vi "Main.vi"() -> ()   [LabVIEW 2014]
uses:
  Enum State Typedef.ctl
  <vilib>/Utility/error.llb/DialogType.ctl
  <vilib>/_DAQmxBase/Internals/DAQmxBase Create Channel (AI-Voltage-Basic).vi
  <vilib>/_DAQmxBase/Internals/DAQmxBase Timing (Sample Clock).vi
  <vilib>/_DAQmxBase/Internals/DAQmxBase Read (Analog 2D DBL NChan NSamp).vi
  <vilib>/Utility/file.llb/Write To Spreadsheet File (DBL).vi
panel:
  out "size(s) 2":i32
  out "State":T1
  in  "Clear Display":bool
  in  "Preview Button":bool
  out "size(s)":i32
  in  "pH":dbl
  in  "Conductivity (mS)":dbl
  out "Iterations Recorded":i32
  in  "Recording Time (seconds)":dbl
  in  "Sample Rate":i32=1000
  in  "physical channels":tag
  in  "Stop Button":bool
  out "Waveform Chart":waveform(dbl)(graph)
  in  "High Pass Filter":enum16{"500", "1k", "5k", "10k", "20k"}(ring)
  in  "Low Pass Filter":enum16{"0.1", "1.0", "10", "100", "300"}(ring)
  in  "Gain":enum16{"x100", "x1000", "x10k"}(ring)
  in  "Notch Filter":bool
  in  "Amplifier Model":u16(ring) items=["Select a Model", "AM 1700", "BMA 200"]
  in  "AC/DC Switch":bool
  in  "Temperature (deg C)":dbl
  in  "User Comments":string
  out "Start Time hr/min":string
  out "Date mm/dd/yy":string
  in  "Species":string
  in  "Exit Button":bool
  in  "Record Button":bool
  # "MSU EFISH Lab Single Channel Electronic Pulse Recorder"
  # "Must enter numbers into here before you run"
  # "Blue for On\nOrange for Off"
  # "DC"
  # "AC"
  # "Blue for AC and Orange for DC"
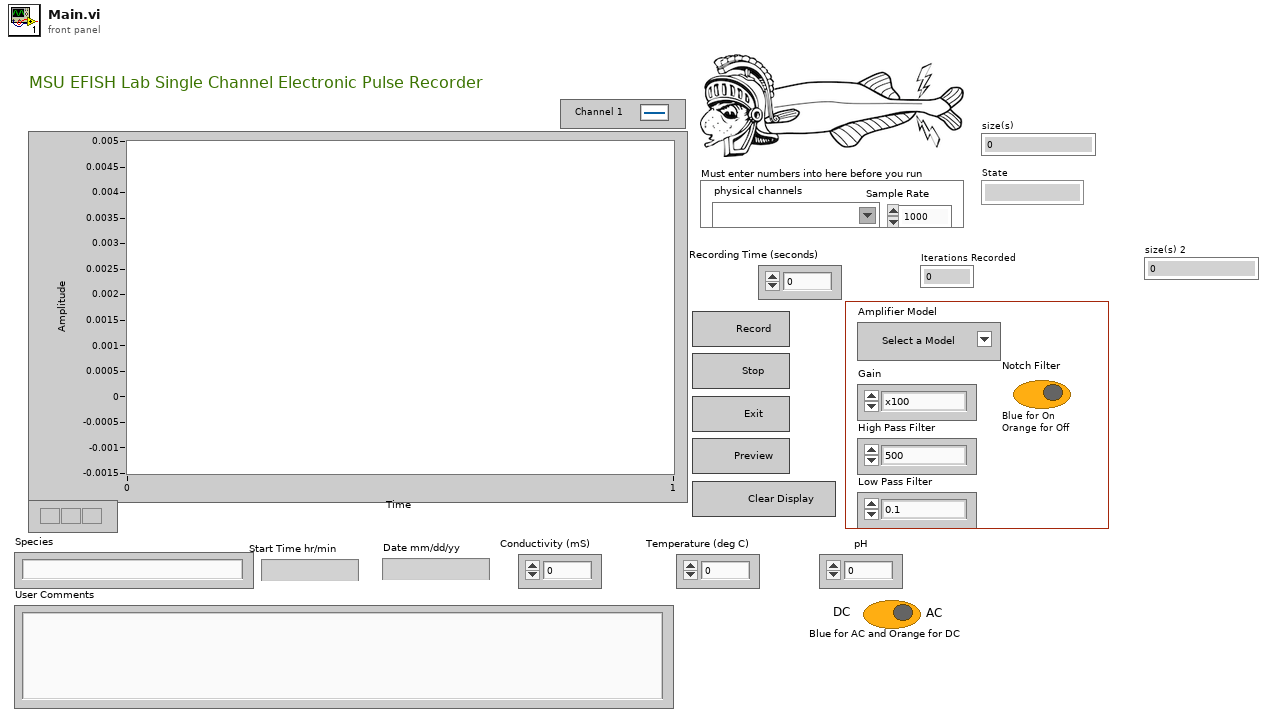
[diagram p1: front panel]
types:
  T1 = typedef "Enum State Typedef.ctl" = enum16{"", "Prepreview Handling", "Clear Display", "Preview Data", "Stop", "Exit", "Record", "Create File"}
  T2 = typedef "DialogType.ctl" = u16
  T3 = cluster{"High Pass Filter":enum16{"500", "1k", "5k", "10k", "20k"}, "Gain":enum16{"x100", "x1000", "x10k"}, "Low Pass Filter":enum16{"0.1", "1.0", "10", "100", "300"}, "Amplifier Model":u16, "Notch Filter":bool, "AC/DC Switch":bool, "Temperature (deg C)":dbl, "Conductivity (mS)":dbl, "pH":dbl, "User Comments":string, "Species":string}
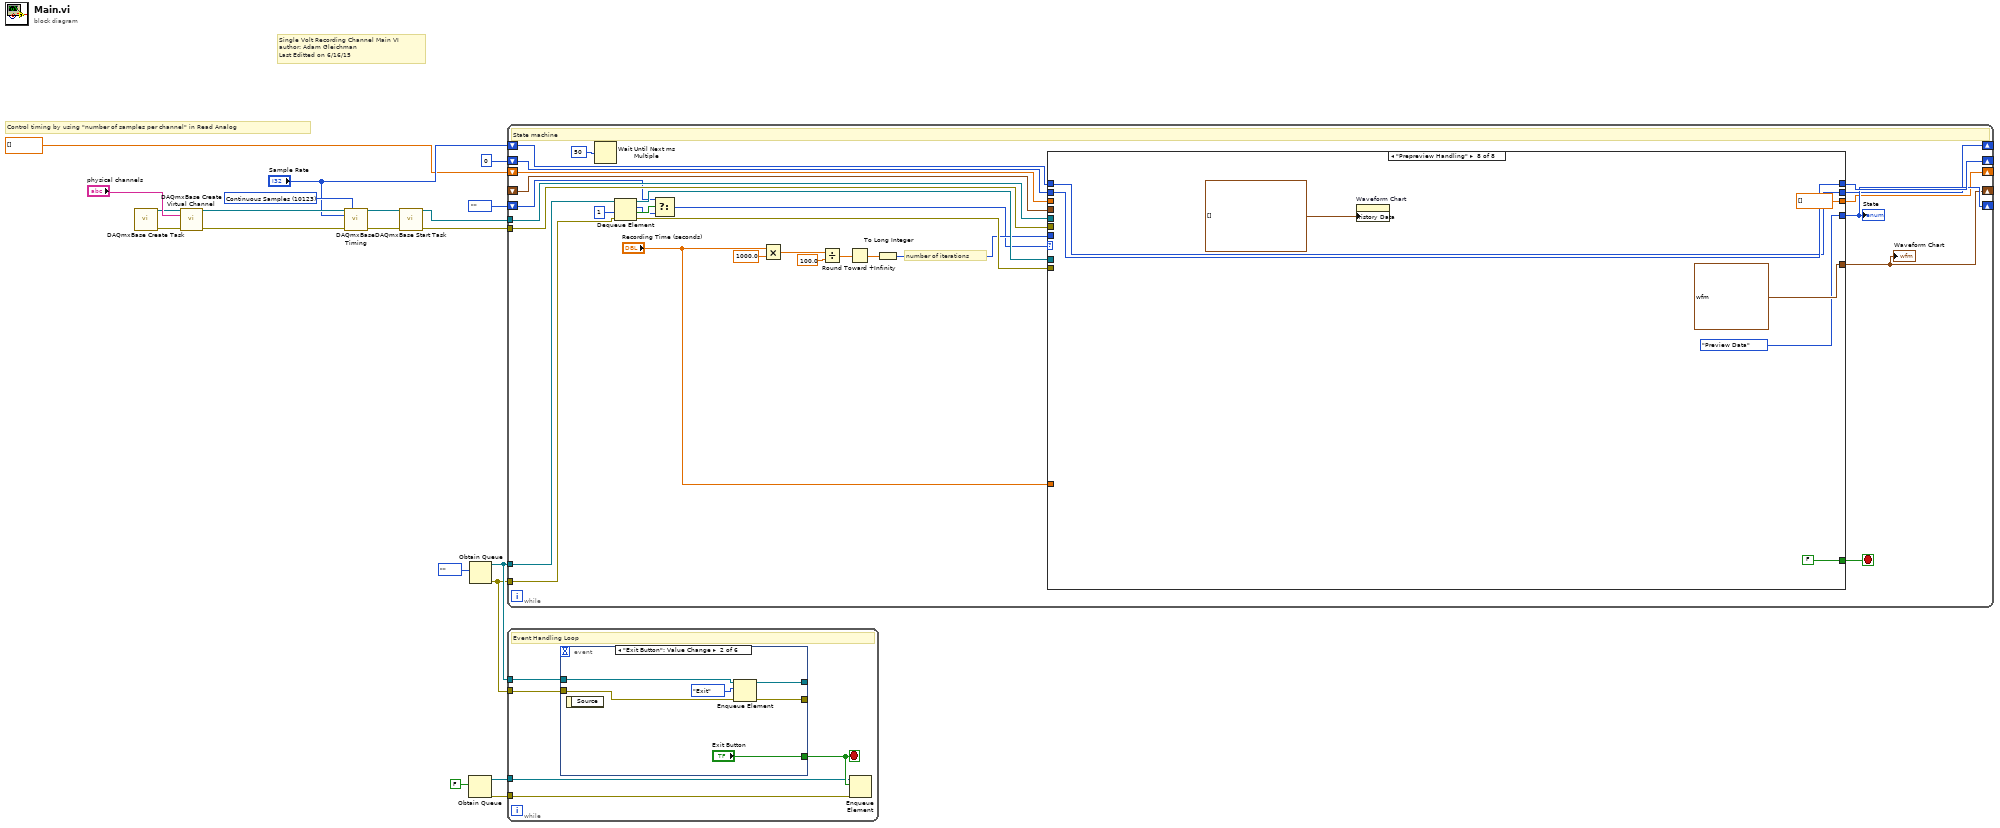
[diagram p0: block diagram]
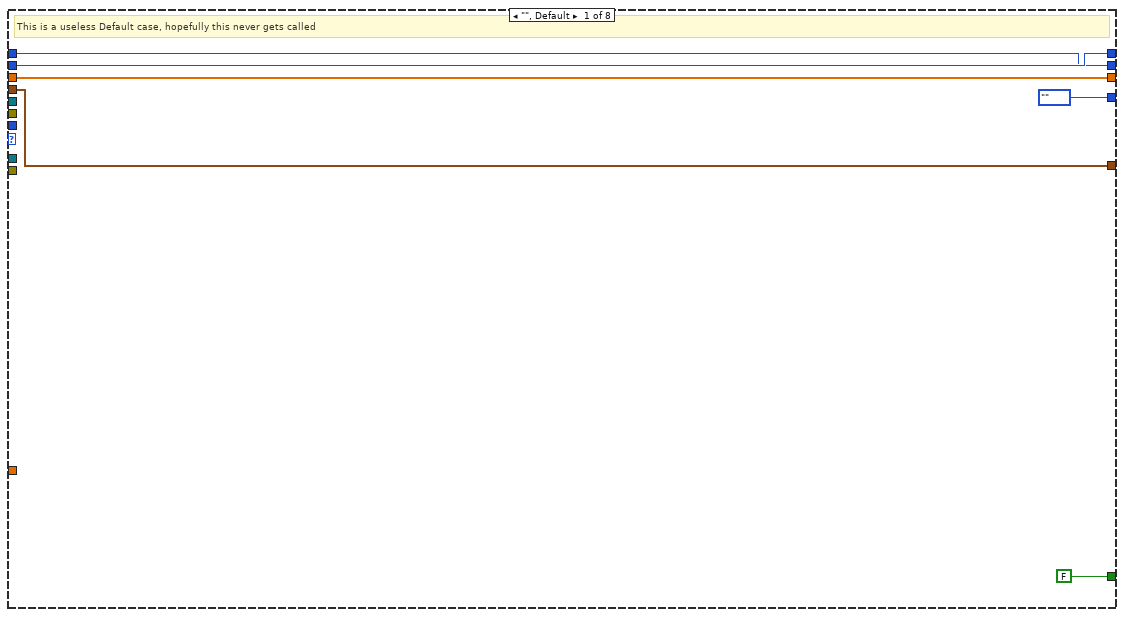
[diagram p2: hidden frame]
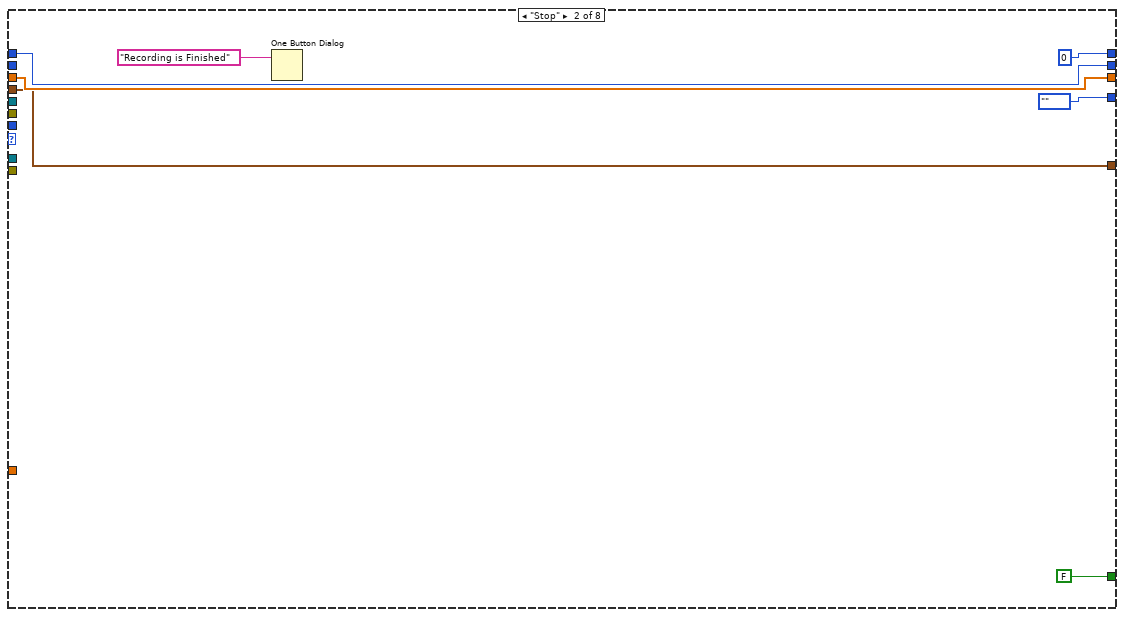
[diagram p3: hidden frame]
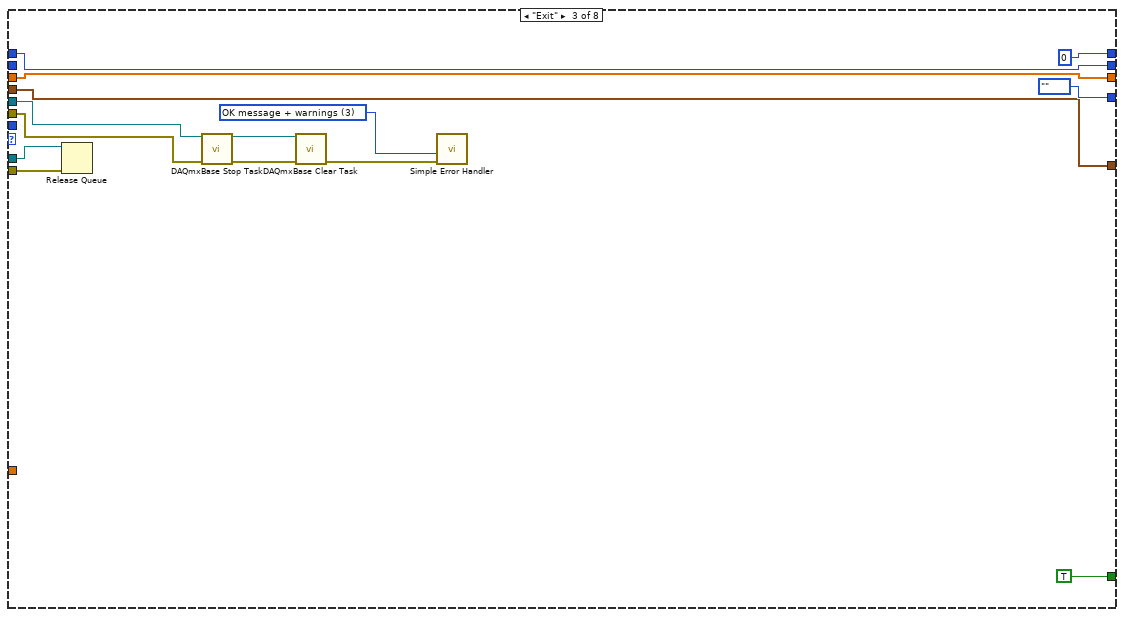
[diagram p4: hidden frame]
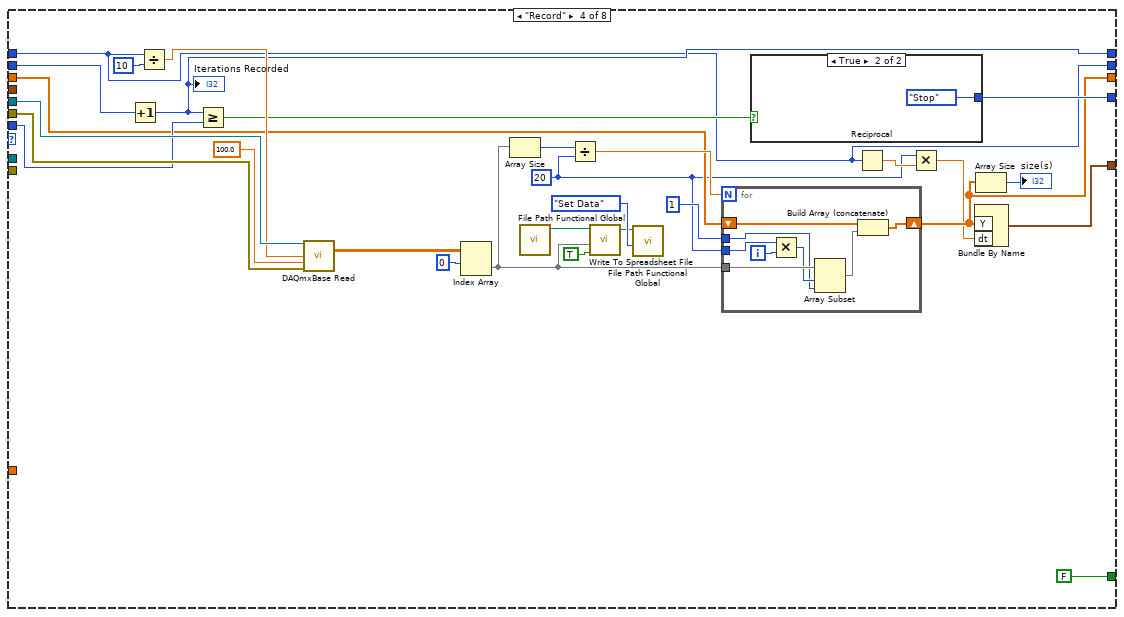
[diagram p5: hidden frame]
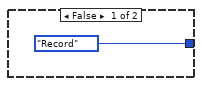
[diagram p6: hidden frame]
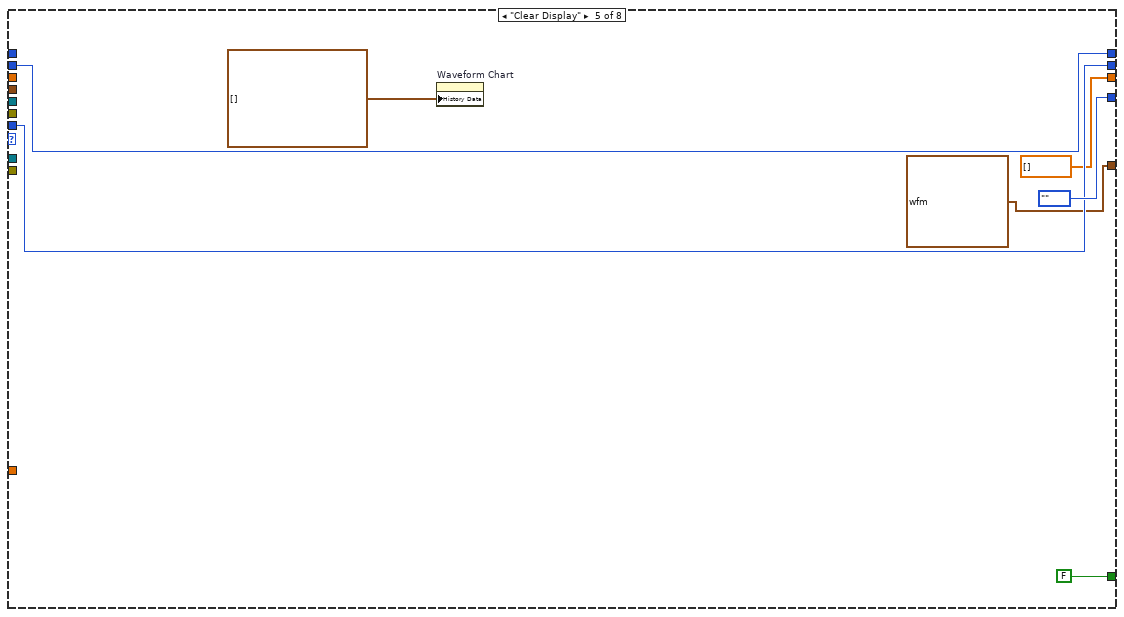
[diagram p7: hidden frame]
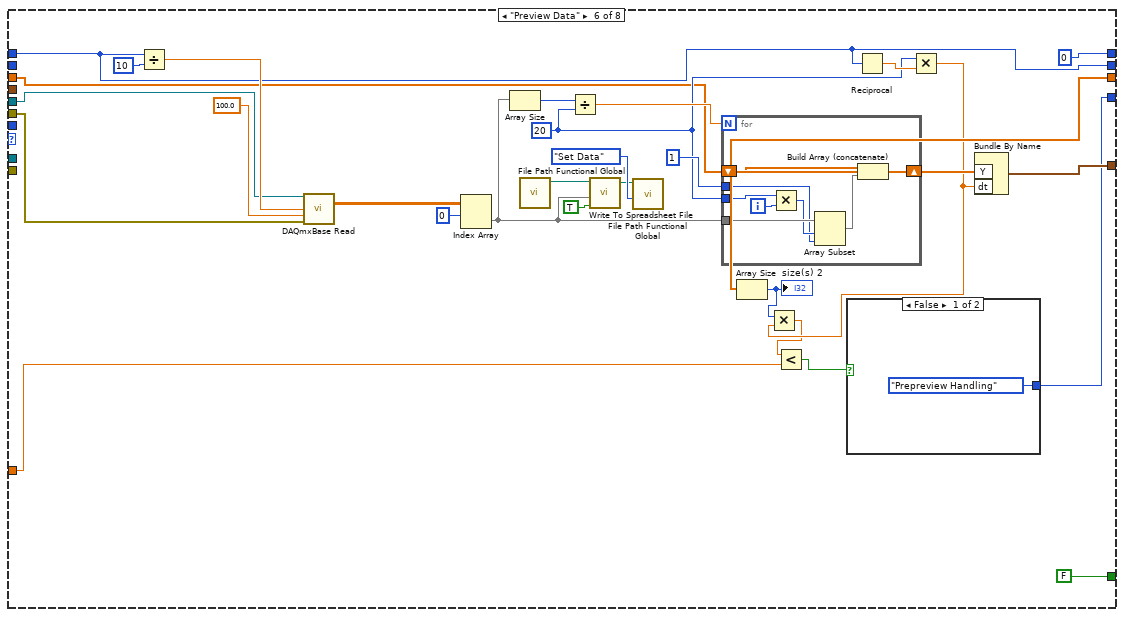
[diagram p8: hidden frame]
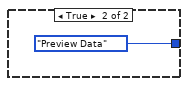
[diagram p9: hidden frame]
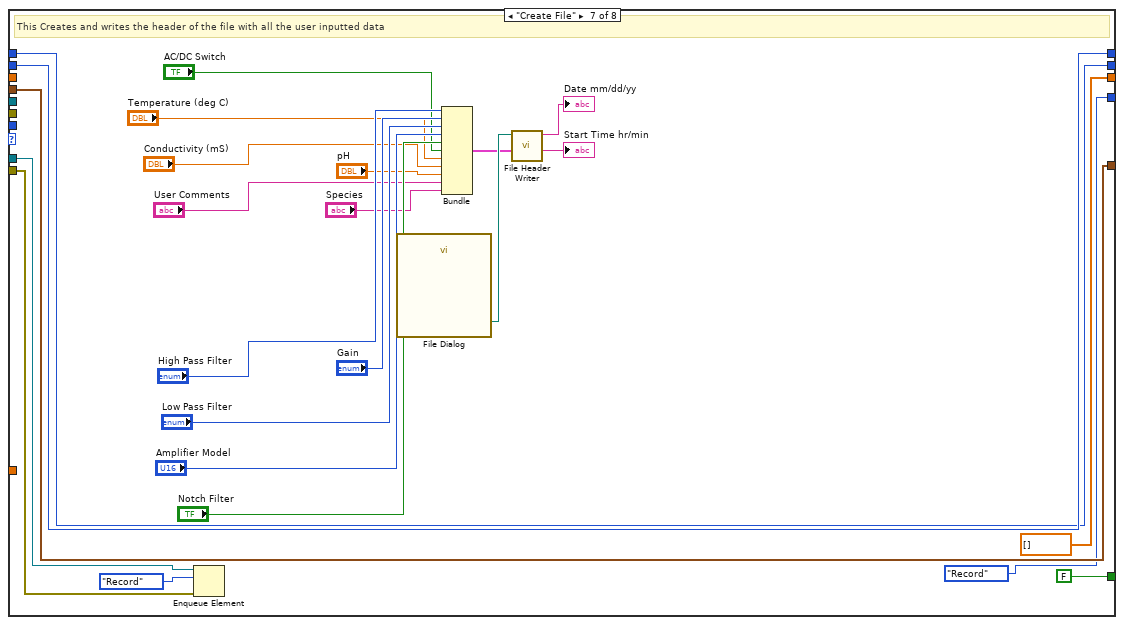
[diagram p10: hidden frame]
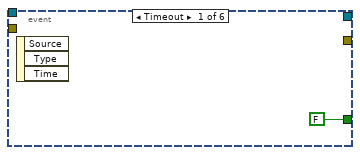
[diagram p11: hidden frame]
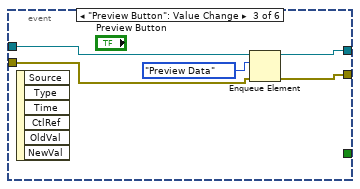
[diagram p12: hidden frame]
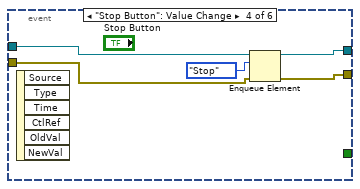
[diagram p13: hidden frame]
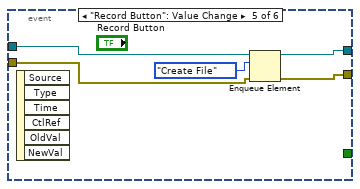
[diagram p14: hidden frame]
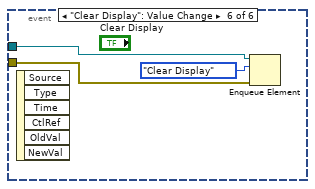
[diagram p15: hidden frame]
diagram:
  w12 = 10123 items=["Finite Samples"=10178, "Continuous Samples"=10123, "Hardware Timed Single Point"=12522] ("sample mode")
  # "Single Volt Recording Channel Main VI\nauthor: Adam Gleichman\nLast Editted on 6/16/15"
  # "Control timing by using \"number of samples per channel\" in Read Analog"
  n1 = call <vilib>:"DAQmxBase Create Task.vi"() -> ("task out"=w16:refnum<k21>, "error out"=w15:errorcluster)  [unwired: 14 in]
  n2 = call-poly <vilib>:"DAQmxBase Create Virtual Channel.vi"("task in"=w16, "physical channels"="physical channels", "error in"=w15) -> ("task out"=w14:refnum<k21>, "error out"=w13:errorcluster)  [unwired: 11 in]
  n3 = call-poly <vilib>:"DAQmxBase Timing.vi"("task/channels in"=w14, "sample mode"=w12, "rate"="Sample Rate", "error in"=w13) -> ("task out"=w11:refnum<k21>, "error out"=w10:errorcluster)  [unwired: 10 in]
  n4 = call <vilib>:"DAQmxBase Start Task.vi"("task/channels in"=w11, "error in"=w10) -> ("task out"=w8:refnum<k21>, "error out"=w9:errorcluster)  [unwired: 12 in]
  n5 = Obtain Queue(element data type=FALSE) -> (queue out=w2:refnum<queue>, error out=w1:errorcluster)  [unwired: 4 in, 1 out]
  n6 = Obtain Queue(element data type=Enum_State_Typedef."" ("State")) -> (queue out=w19:refnum<queue>, error out=w18:errorcluster)  [unwired: 4 in, 1 out]
  n7 = while {
    tunnel: w19 -> [w49]
    tunnel: w18 -> [w48]
    tunnel: w9 -> [w43]
    tunnel: w8 -> [w44]
    shift-right: [w35] -> _
    shift-left: 0 -> [w36]
    shift-right: [w30] -> _
    shift-left: Enum_State_Typedef."" ("State") -> [w32]
    shift-right: [w28] -> _
    shift-left: "Sample Rate" -> [w29]
    shift-right: [w22] -> _
    shift-left: dbl[] [] -> [w25]
    shift-right: [w24] -> _
    shift-left: _ -> [w23]
    stop <- w47 stop-if-true
    # "number of iterations"
    # "State machine"
    n8 = Wait Until Next ms Multiple(millisecond multiple=u32 50) -> ()  [unwired: 1 out]
    n9 = Dequeue Element(queue=w49, timeout in ms (-1)=1, error in (no error)=w48) -> (queue out=w46:refnum<queue>, element=w33:T1, timed out?=w34:bool, error out=w45:errorcluster)
    n10 = Select(t=w32, s=w34, f=w33) -> (s? t:f=w31:T1)
    n11 = Multiply(x="Recording Time (seconds)", y=1000.0) -> (x*y=w41:dbl)
    n12 = Divide(x=w41, y=100.0) -> (x/y=w39:dbl)
    n13 = Round Toward +Infinity(x=w39) -> (ceil(x): smallest int >= x=w38:dbl)
    n14 = To Long Integer(number=w38) -> (32bit integer=w37:i32)
    n15 = case shown="\"Prepreview Handling\"" w31 {
      tunnel: [FALSE FALSE TRUE FALSE FALSE FALSE FALSE FALSE] -> w47
      tunnel: w46 -> [_ _ w69 _ _ _ w185 _]
      tunnel: w45 -> [_ _ w68 _ _ _ w184 _]
      tunnel: w44 -> [_ _ w73 w104 _ w133 _ _]
      tunnel: w43 -> [_ _ w72 w103 _ w132 _ _]
      tunnel: w29 -> [w52 w59 w65 w80 _ w128 w181 w187]
      tunnel: w37 -> [_ _ _ w96 w119 _ _ _]
      tunnel: w36 -> [w54 _ _ w97 w122 _ w182 w188]
      tunnel: [w54 0 0 w91 w122 0 w182 w188] -> w35
      tunnel: [Enum_State_Typedef."" ("State") Enum_State_Typedef."" ("State") Enum_State_Typedef."" ("State") w93 Enum_State_Typedef."" ("State") w130 Enum_State_Typedef."Record" ("State") Enum_State_Typedef."Preview Data" ("State")] -> w30
      tunnel: [w52 w59 w65 w80 w119 w128 w181 w187] -> w28
      tunnel: [w51 w57 w64 w84 dbl[] [] w129 dbl[] [] dbl[] []] -> w22
      tunnel: w25 -> [w51 w57 w64 w83 _ w134 _ _]
      tunnel: [w50 w56 w63 w82 waveform(dbl) {"t0"=timestamp(0 s since 1904-01-01), "dt"=1.0, "Y"=[]} w131 w169 waveform(dbl) {"t0"=timestamp(0 s since 1904-01-01), "dt"=1.0, "Y"=[]}] -> w24
      tunnel: w23 -> [w50 w56 w63 _ _ _ w169 _]
      tunnel: "Recording Time (seconds)" -> [_ _ _ _ _ w126 _ _]
      frame "", Default {
        # "This is a useless Default case, hopefully this never gets called"
      }
      frame "Stop" {
        n16 = One Button Dialog(message="Recording is Finished") -> ()  [unwired: 1 in, 1 out]
      }
      frame "Exit" {
        w70 = T2 3 items=["no dialog", "OK message", "continue or stop message", "OK message + warnings", "continue/stop + warnings"] ("type of dialog (OK msg:1)")
        n17 = Release Queue(queue=w69, error in (no error)=w68) -> ()  [unwired: 1 in, 3 out]
        n18 = call <vilib>:"DAQmxBase Stop Task.vi"("task/channels in"=w73, "error in"=w72) -> ("task out"=w75:refnum<k21>, "error out"=w74:errorcluster)  [unwired: 12 in]
        n19 = call <vilib>:"DAQmxBase Clear Task.vi"("task in"=w75, "error in"=w74) -> ("error out"=w71:errorcluster)  [unwired: 13 in]
        n20 = call <vilib>:"Simple Error Handler.vi"("type of dialog (OK msg:1)"=w70, "error in (no error)"=w71) -> ()  [unwired: 3 in, 5 out]
      }
      frame "Record" {
        w78 = 20 ("y")
        n21 = Increment(x=w97) -> (x+1=w91:i32)
        "Iterations Recorded" <- w91
        n22 = Divide(x=w80, y=10) -> (x/y=w94:dbl)
        n23 = Greater Or Equal?(x=w91, y=w96) -> (x >= y?=w92:bool)
        n24 = call-poly <vilib>:"DAQmxBase Read.vi"("task/channels in"=w104, "number of samples per channel"=w94, "timeout"=100.0, "error in"=w103) -> ("data"=w89:dbl[][])  [unwired: 9 in, 2 out]
        n25 = Index Array(array=w89, index (row)=0) -> (element=w81:dbl[])  [unwired: 1 in]
        n26 = Array Size(array=w81) -> (size(s)=w88:i32)
        n27 = call "File Path Functional Global.vi"() -> ("File Path Output"=w101:path)  [unwired: 11 in]
        n28 = Divide(x=w88, y=w78) -> (x/y=w87:dbl)
        n29 = call-poly <vilib>:"Write To Spreadsheet File.vi"("append to file? (new file:F)"=TRUE, "1D data"=w81, "file path (dialog if empty)"=w101) -> ("new file path (Not A Path if cancelled)"=w99:path)  [unwired: 5 in]
        n30 = call "File Path Functional Global.vi"("Enum"=enum16{"Get Data", "Set Data"}."Set Data", "File Path Control"=w99) -> ()  [unwired: 9 in, 1 out]
        n31 = for {
          N: w87 -> [_]
          shift-right: [w106] -> w84
          shift-left: w83 -> [w108]
          tunnel: w81 -> [w113]
          tunnel: w78 -> [w111]
          tunnel: 1 ("y") -> [w109]
          i -> [w112]
          n32 = Multiply(x=w111, y=w112) -> (x*y=w110:i32)
          n33 = Array Subset(array=w113, index=w110, length=w109) -> (w107:dbl[])
          n34 = Build Array (concatenate)(w108, w107) -> (w106:dbl[])
        }
        n35 = case shown="True" w92 {
          tunnel: [Enum_State_Typedef."Record" ("State") Enum_State_Typedef."Stop" ("State")] -> w93
          frame False {
          }
          frame True {
          }
        }
        n36 = Reciprocal(x=w80) -> (1/x=w79:dbl)
        n37 = Multiply(x=w78, y=w79) -> (x*y=w77:dbl)
        n38 = Bundle By Name("Y"=w84, "dt"=w77) -> (w82:waveform(dbl))  [unwired: 1 in]
        n39 = Array Size(array=w84) -> (size(s)=→"size(s)":i32)
      }
      frame "Clear Display" {
        n40 = property on="Waveform Chart" class="WFChart (strict)"("History Data"=waveform(dbl)[] []) -> ()  [unwired: 2 in, 2 out]
      }
      frame "Preview Data" {
        w135 = 20 ("y")
        n41 = Divide(x=w128, y=10) -> (x/y=w143:dbl)
        n42 = call-poly <vilib>:"DAQmxBase Read.vi"("task/channels in"=w133, "number of samples per channel"=w143, "timeout"=100.0, "error in"=w132) -> ("data"=w141:dbl[][])  [unwired: 9 in, 2 out]
        n43 = Index Array(array=w141, index (row)=0) -> (element=w137:dbl[])  [unwired: 1 in]
        n44 = Array Size(array=w137) -> (size(s)=w140:i32)
        n45 = call "File Path Functional Global.vi"() -> ("File Path Output"=w148:path)  [unwired: 11 in]
        n46 = Divide(x=w140, y=w135) -> (x/y=w139:dbl)
        n47 = call-poly <vilib>:"Write To Spreadsheet File.vi"("append to file? (new file:F)"=TRUE, "1D data"=w137, "file path (dialog if empty)"=w148) -> ("new file path (Not A Path if cancelled)"=w146:path)  [unwired: 5 in]
        n48 = call "File Path Functional Global.vi"("Enum"=enum16{"Get Data", "Set Data"}."Set Data", "File Path Control"=w146) -> ()  [unwired: 9 in, 1 out]
        n49 = for {
          N: w139 -> [_]
          shift-right: [w154] -> w129
          shift-left: w134 -> [w156]
          tunnel: w137 -> [w161]
          tunnel: w135 -> [w159]
          tunnel: 1 ("y") -> [w157]
          i -> [w160]
          n50 = Multiply(x=w159, y=w160) -> (x*y=w158:i32)
          n51 = Array Subset(array=w161, index=w158, length=w157) -> (w155:dbl[])
          n52 = Build Array (concatenate)(w156, w155) -> (w154:dbl[])
        }
        n53 = Array Size(array=w129) -> (size(s)=w125:i32)
        "size(s) 2" <- w125
        n54 = Reciprocal(x=w128) -> (1/x=w136:dbl)
        n55 = Multiply(x=w135, y=w136) -> (x*y=w124:dbl)
        n56 = Multiply(x=w125, y=w124) -> (x*y=w123:dbl)
        n57 = Less?(x=w123, y=w126) -> (x < y?=w127:bool)
        n58 = case shown="False" w127 {
          tunnel: [Enum_State_Typedef."Prepreview Handling" ("State") Enum_State_Typedef."Preview Data" ("State")] -> w130
          frame False {
          }
          frame True {
          }
        }
        n59 = Bundle By Name("Y"=w129, "dt"=w124) -> (w131:waveform(dbl))  [unwired: 1 in]
      }
      frame "Create File" {
        # "This Creates and writes the header of the file with all the user inputted data"
        n60 = Enqueue Element(queue=w185, element=Enum_State_Typedef."Record", error in (no error)=w184) -> ()  [unwired: 1 in, 3 out]
        n61 = call "File Dialog"() -> ("selected path"=w166:path)  [unwired: 12 in, 3 out]
        n62 = Bundle("High Pass Filter"="High Pass Filter", "Gain"="Gain", "Low Pass Filter"="Low Pass Filter", "Amplifier Model"="Amplifier Model", "Notch Filter"="Notch Filter", "AC/DC Switch"="AC/DC Switch", "Temperature (deg C)"="Temperature (deg C)", "Conductivity (mS)"="Conductivity (mS)", "pH"="pH", "User Comments"="User Comments", "Species"="Species") -> (w165:T3)  [unwired: 1 in]
        n63 = call "File Header Writer.vi"("Data Cluster"=w165, "File Path"=w166) -> ("Start Time hr/min"=→"Start Time hr/min":string, "Date mm/dd/yy"=→"Date mm/dd/yy":string)  [unwired: 8 in]
      }
      frame "Prepreview Handling" {
        n64 = property on="Waveform Chart" class="WFChart (strict)"("History Data"=waveform(dbl)[] []) -> ()  [unwired: 2 in, 2 out]
      }
    }
    "Waveform Chart" <- w24
    "State" <- w30
  }
  n65 = while {
    tunnel: w19 -> [w197]
    tunnel: w18 -> [w196]
    tunnel: w2 -> [w194]
    tunnel: w1 -> [w193]
    stop <- w195 stop-if-true
    # "Event Handling Loop"
    n66 = event shown="[1] \"Exit Button\": Value Change" {
      selector: _ -> [_ _ _ _ _ _]
      dyn-events: _ -> [_ _ _ _ _ _]
      timeout: _ -> [_ _ _ _ _ _]
      tunnel: [FALSE ("Exit Button") "Exit Button" _ _ _ _] -> w195
      tunnel: w197 -> [_ w203 w209 w214 w219 w222]
      tunnel: w196 -> [_ w202 w208 w213 w218 w221]
      tunnel: [_ w201 w206 w211 w216 _] -> _
      tunnel: [_ w200 w205 w212 w217 _] -> _
      event Timeout {
        n67 = event-data() -> ()  [unwired: 1 in, 3 out]
      }
      event "Exit Button": Value Change {
        n68 = event-data() -> ()  [unwired: 1 in, 1 out]
        n69 = Enqueue Element(queue=w203, element=Enum_State_Typedef."Exit", error in (no error)=w202) -> (queue out=w201:refnum<queue>, error out=w200:errorcluster)  [unwired: 1 in, 1 out]
      }
      event "Preview Button": Value Change {
        n70 = event-data() -> ()  [unwired: 1 in, 6 out]
        n71 = Enqueue Element(queue=w209, element=Enum_State_Typedef."Preview Data", error in (no error)=w208) -> (queue out=w206:refnum<queue>, error out=w205:errorcluster)  [unwired: 1 in, 1 out]
      }
      event "Stop Button": Value Change {
        n72 = event-data() -> ()  [unwired: 1 in, 6 out]
        n73 = Enqueue Element(queue=w214, element=Enum_State_Typedef."Stop", error in (no error)=w213) -> (queue out=w211:refnum<queue>, error out=w212:errorcluster)  [unwired: 1 in, 1 out]
      }
      event "Record Button": Value Change {
        n74 = event-data() -> ()  [unwired: 1 in, 6 out]
        n75 = Enqueue Element(queue=w219, element=Enum_State_Typedef."Create File", error in (no error)=w218) -> (queue out=w216:refnum<queue>, error out=w217:errorcluster)  [unwired: 1 in, 1 out]
      }
      event "Clear Display": Value Change {
        n76 = event-data() -> ()  [unwired: 1 in, 6 out]
        n77 = Enqueue Element(queue=w222, element=Enum_State_Typedef."Clear Display", error in (no error)=w221) -> ()  [unwired: 1 in, 3 out]
      }
    }
    n78 = Enqueue Element(queue=w194, element=w195, error in (no error)=w193) -> ()  [unwired: 1 in, 3 out]
  }
